vi "Accelerometer.vi"() -> ()   [LabVIEW 2012]
uses:
  <vilib>/eio/EIONode/EIONode.xnode
  <vilib>/rvi/eio/common/nirviEmuTemplateMethod_errors.vi
  <vilib>/eio/EIOPropertyNode/EIOPropertyNode.xnode
  <vilib>/LabVIEW Targets/FPGA/cRIO/shared/nicrio_ModuleControls/nicrio_cRIO-9234_DataRatesRing2.ctl
  <vilib>/rvi/eio/common/nirviEmuTemplatePropertyGet_errors.vi
  <vilib>/rvi/eio/common/nirviEmuTemplatePropertyGet_noerrors.vi
  <vilib>/rvi/eio/common/nirviEmuTemplatePropertySet_errors.vi
  <vilib>/rvi/eio/common/nirviEmuTemplatePropertySet_noerrors.vi
panel:
  in  "Acceleration Threshold":fxp<+/-,24,4> format="%.22g"
  in  "Fan Speed Control":fxp<+/-,20,5> format="%_6g"
  in  "Stop":bool
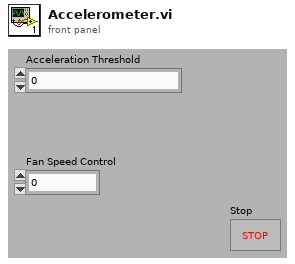
[diagram p1: front panel]
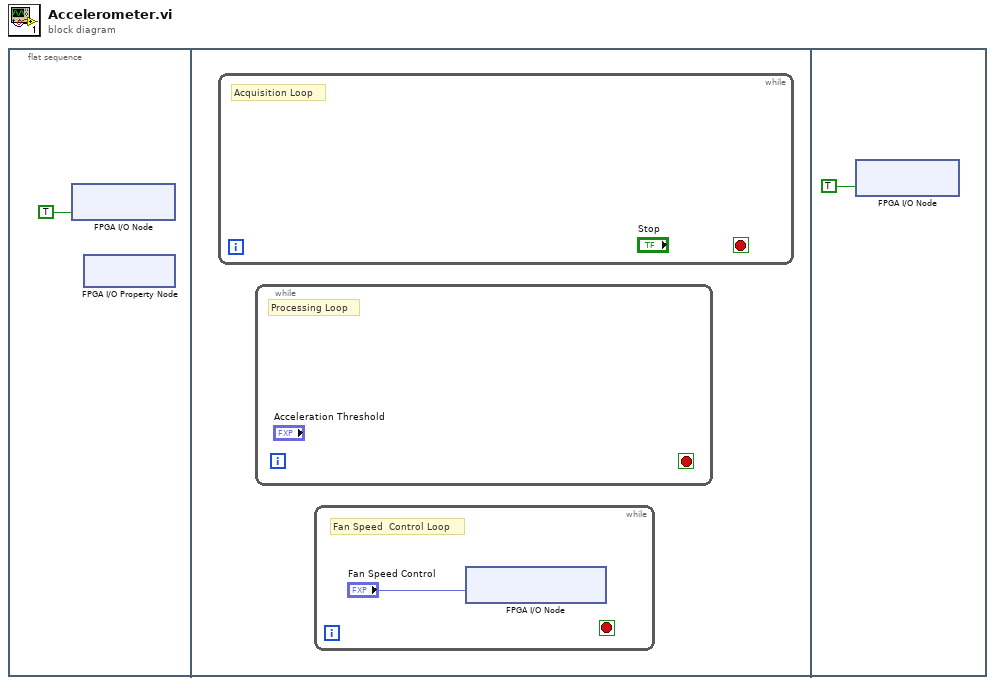
[diagram p0: block diagram]
diagram:
  n1 = flat-sequence {
    frame #0 {
      n2 = xnode "FPGA I/O Node"("Mod2/Start"=TRUE) -> ()  [unwired: 1 in, 1 out]
      n3 = xnode "FPGA I/O Property Node"() -> ()  [unwired: 2 in, 1 out]
    }
    frame #1 {
      n4 = while {
        stop <- _ stop-if-true
        # "Acquisition Loop"
      }
      n5 = while {
        stop <- _ stop-if-true
        # "Processing Loop"
      }
      n6 = while {
        stop <- _ stop-if-true
        # "Fan Speed  Control Loop"
        n7 = xnode "FPGA I/O Node"("Fan Speed Control"="Fan Speed Control") -> ()  [unwired: 1 in, 1 out]
      }
    }
    frame #2 {
      n8 = xnode "FPGA I/O Node"("Mod2/Stop"=TRUE ("Mod2/Start")) -> ()  [unwired: 1 in, 1 out]
    }
  }
